vi "timestamps.vi"() -> ()   [LabVIEW 2011]
panel:
  out "Channels":i8[](array[numeric])
  out "Timestamps":i64[](array[numeric])
  out "Data Lost":bool
  out "Error Out":errorcluster
  out "Timestamp Count":i32
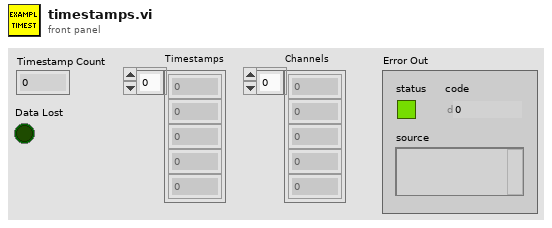
[diagram p1: front panel]
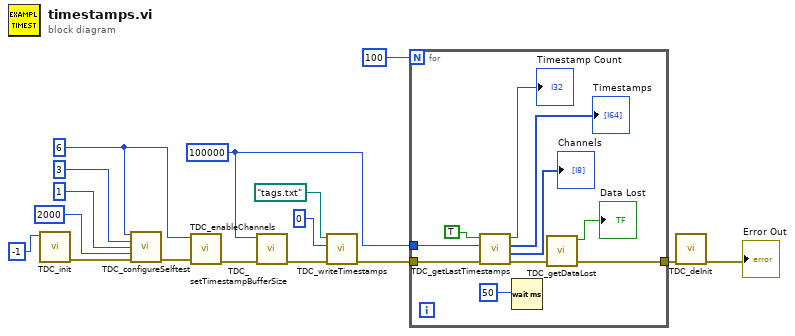
[diagram p0: block diagram]
diagram:
  w1 = 100000
  w7 = 6
  n1 = call "TDC_init.vi"("Device ID"=-1) -> ("Error Out"=w15:errorcluster)  [unwired: 10 in]
  n2 = call "TDC_configureSelftest.vi"("Channel Mask"=w7, "Period [5ns]"=3, "Burst Size"=1, "Burst Distance [20 ns]"=2000, "Error In"=w15) -> ("Error Out"=w8:errorcluster)  [unwired: 10 in]
  n3 = call "TDC_enableChannels.vi"("Error In"=w8, "Channel Mask"=w7) -> ("Error Out"=w6:errorcluster)  [unwired: 9 in]
  n4 = call "TDC_setTimestampBufferSize.vi"("Error In"=w6, "Buffer Size"=w1) -> ("Error Out"=w5:errorcluster)  [unwired: 9 in]
  n5 = call "TDC_writeTimestamps.vi"("Error In"=w5, "Data Format"=0, "Path"=path "tags.txt") -> ("Error Out"=w10:errorcluster)  [unwired: 8 in]
  n6 = for {
    N: 100 -> [_]
    tunnel: w10 -> [w25]
    tunnel: [w23] -> w9
    tunnel: w1 -> [w20]
    n7 = call "TDC_getLastTimestamps.vi"("Error In"=w25, "Buffer Size"=w20, "Reset"=TRUE) -> ("Error Out"=w22:errorcluster, "Channel Numbers"=→"Channels":i8[], "Timestamps"=→"Timestamps":i64[], "Valid Data"=→"Timestamp Count":i32)  [unwired: 5 in]
    n8 = Wait (ms)(milliseconds to wait=50) -> ()  [unwired: 1 out]
    n9 = call "TDC_getDataLost.vi"("Error In"=w22) -> ("Error Out"=w23:errorcluster, "Data Loss"=→"Data Lost":bool)  [unwired: 9 in]
  }
  n10 = call "TDC_deInit.vi"("Error In"=w9) -> ("Error Out"=→"Error Out":errorcluster)  [unwired: 10 in]
